vi "Stop Core.vi"(10 "final error code":i32, 11 "Chat Window in":refnum<class "Chat Window.lvclass">) -> (3 "Chat Window out":refnum<class "Chat Window.lvclass">)   [LabVIEW 2020, in "Chat Window.lvlib" / "Chat Window.lvclass"]
doc: "(<B>Filename</B>: Actor Framework.lvlib:Actor.lvclass:Stop Core.vi)\n\nDefines what the actor does before it stops. Use the <B>final error code</B> input to determine whether the actor shut down in response to an error.\n\nBy default, this method does nothing. A descendant class may override it to define behavior, such as shutting down any processes the actor initiated in its override of the Actor Core method."
uses:
  Chat Window.lvclass
  <vilib>/ActorFramework/Actor/Actor.lvclass
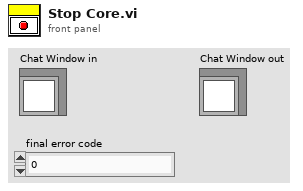
[diagram p1: front panel]
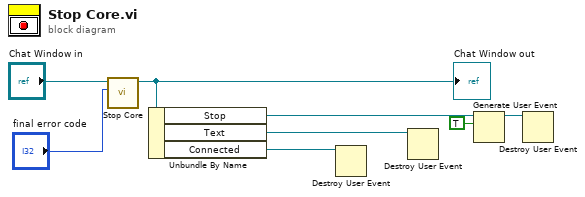
[diagram p0: block diagram]
diagram:
  n1 = call-parent "Stop Core.vi"("final error code"="final error code", "Actor in"="Chat Window in") -> ("Actor out"=w6:refnum<class "Chat Window.lvclass">)  [unwired: 9 in]
  "Chat Window out" <- w6
  n2 = Unbundle By Name(w6) -> ("Stop"=w5:refnum<user-event>, "Text"=w3:refnum<user-event>, "Connected"=w1:refnum<user-event>)
  n3 = Destroy User Event(user event=w1) -> ()  [unwired: 1 in, 1 out]
  n4 = Destroy User Event(user event=w3) -> ()  [unwired: 1 in, 1 out]
  n5 = Generate User Event(user event=w5, event data cluster=TRUE ("event data")) -> (user event out=w2:refnum<user-event>)  [unwired: 2 in, 1 out]
  n6 = Destroy User Event(user event=w2) -> ()  [unwired: 1 in, 1 out]
